vi "standupRoutine2.vi"(10 "x":dbl, 11 "theta":dbl) -> (3 "force":dbl)   [LabVIEW 2013]
uses:
  <vilib>/addons/control/pid/pid.llb/PID Control Input Filter (DBL).vi
  <vilib>/addons/control/pid/pid.llb/PID (DBL).vi
  <vilib>/addons/control/pid/NI_PID_pid.lvlib
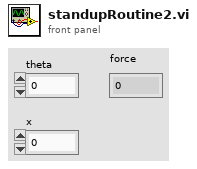
[diagram p1: front panel]
types:
  T1 = cluster{"proportional gain (Kc)":dbl, "integral time (Ti, min)":dbl, "derivative time (Td, min)":dbl}
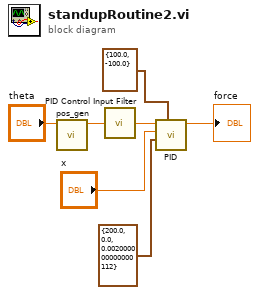
[diagram p0: block diagram]
diagram:
  n1 = call "pos_gen.vi"("theta"="theta") -> ("x_d"=w2:dbl)  [unwired: 10 in]
  n2 = call-poly <vilib>:"PID Control Input Filter.vi"("input"=w2) -> ("output"=w1:dbl)  [unwired: 4 in]
  n3 = call-poly <vilib>:"PID.vi"("output range"=cluster{"output high":dbl, "output low":dbl} {"output high"=100.0, "output low"=-100.0}, "PID gains"=T1 {"proportional gain (Kc)"=200.0, "integral time (Ti, min)"=0.0, "derivative time (Td, min)"=0.002000000000000112}, "process variable"="x", "setpoint"=w1) -> ("output"=→"force":dbl)  [unwired: 6 in, 1 out]
